vi "BuildGmaterial.vi"(1 "texture":string, 2 "link color":u32(colorbox)=11812608) -> (0 "sdf":string="<material>\n  <ambient> 0.705882 0.247059 0.000000 1.000000</ambient>\n</material>\n")   [LabVIEW 2012]
panel:
  in  "alpha":dbl=1.0
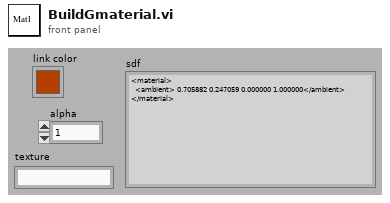
[diagram p1: front panel]
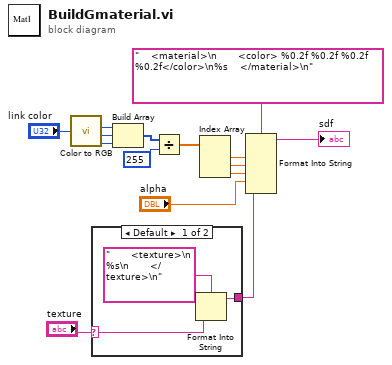
[diagram p0: block diagram]
diagram:
  n1 = call <vilib>:"Color to RGB.vi"("Color"="link color") -> ("R"=w5:u8, "G"=w7:u8, "B"=w6:u8)  [unwired: 1 out]
  n2 = case shown="Default" "texture" {
    selector: "texture" -> [w18 w19]
    tunnel: [w17 w19] -> w1
    frame Default {
      n3 = Format Into String(format string="       <texture>\n          %s\n       </texture>\n", w18) -> (resulting string=w17:string)  [unwired: 2 in, 1 out]
    }
    frame "" {
    }
  }
  n4 = Build Array(w5, w7, w6) -> (w8:u8[])
  n5 = Divide(x=w8, y=u8 255 ("element")) -> (x/y=w12:dbl[])
  n6 = Index Array(array=w12) -> (element #1=w11:dbl, element #2=w13:dbl, element #3=w14:dbl)  [unwired: 3 in]
  n7 = Format Into String(format string="    <material>\n       <color> %0.2f %0.2f %0.2f %0.2f</color>\n%s    </material>\n", w11, w13, w14, "alpha", w1) -> (resulting string=→"sdf":string)  [unwired: 2 in, 1 out]
